vi "init_panel.vi"(6 "Run":refnum<vi>, 7 "Succesfull Run":refnum<vi>, 8 "Parameters Tree":refnum<vi>, 9 "Plot Tree":refnum<vi>, 10 "Spec File Loaded?":refnum<vi>, 11 "Vali File Loaded?":refnum<vi>) -> ()   [LabVIEW 2019]
uses:
  Biogas_LabView_Wrapper/lib/libBioGasLabViewWrapper.so
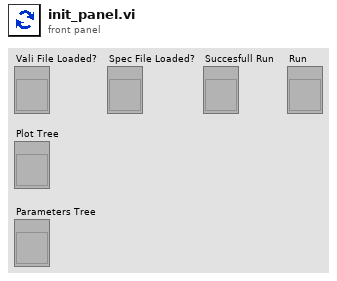
[diagram p1: front panel]
types:
  T1 = enum8{"Enabled", "Disabled", "Disabled and Grayed Out"}
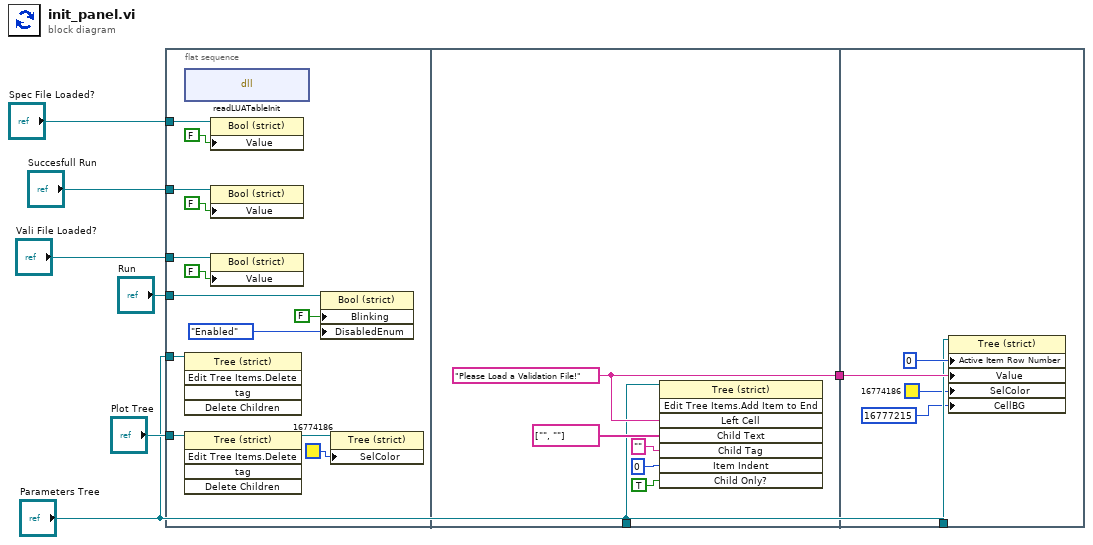
[diagram p0: block diagram]
diagram:
  n1 = flat-sequence {
    tunnel: "Vali File Loaded?" -> [w19]
    tunnel: "Plot Tree" -> [w18]
    tunnel: "Parameters Tree" -> [w17]
    tunnel: "Spec File Loaded?" -> [w16]
    tunnel: "Succesfull Run" -> [w14]
    tunnel: "Run" -> [w12]
    tunnel: [w23] -> w7
    tunnel: "Parameters Tree" -> [w21]
    tunnel: w7 -> [w30]
    tunnel: "Parameters Tree" -> [w29]
    frame #0 {
      n2 = dll-call lib="home/paul/Schreibtisch/Biogas_LabView_Wrapper/lib/libBioGasLabViewWrapper.so" fn="readLUATableInit"() -> ()  [unwired: 4 in, 2 out]
      n3 = invoke on="Invoke Node" class="Tree (strict)" method="Edit Tree Items.Delete"(reference=w17) -> ()  [unwired: 4 in, 5 out]
      n4 = invoke on="Invoke Node" class="Tree (strict)" method="Edit Tree Items.Delete"(reference=w18) -> (reference out=w9:refnum<vi>)  [unwired: 4 in, 4 out]
      n5 = property class="Bool (strict)"(reference=w16, "Value"=FALSE) -> ()  [unwired: 1 in, 2 out]
      n6 = property class="Bool (strict)"(reference=w14, "Value"=FALSE) -> ()  [unwired: 1 in, 2 out]
      n7 = property class="Bool (strict)"(reference=w19, "Value"=FALSE ("Vali File Loaded")) -> ()  [unwired: 1 in, 2 out]
      n8 = property class="Bool (strict)"(reference=w12, "Blinking"=FALSE, "DisabledEnum"=T1."Enabled" ("Disabled")) -> ()  [unwired: 1 in, 2 out]
      n9 = property class="Tree (strict)"(reference=w9, "SelColor"=u32 16774186) -> ()  [unwired: 1 in, 2 out]
    }
    frame #1 {
      w23 = "Please Load a Validation File!" ("Parent Tag")
      n10 = invoke on="Invoke Node" class="Tree (strict)" method="Edit Tree Items.Add Item to End"(reference=w21, "Left Cell"=w23, "Child Text"=string[] ["", ""], "Child Tag"="", "Item Indent"=0 ("New Item Indentation"), "Child Only?"=TRUE) -> ()  [unwired: 2 in, 8 out]
    }
    frame #2 {
      n11 = property on="Property Node" class="Tree (strict)"(reference=w29, "Active Item Row Number"=0 ("Active Item:Row Number"), "Value"=w30, "SelColor"=u32 16774186, "CellBG"=u32 16777215 ("Active Cell:Background Color")) -> ()  [unwired: 1 in, 2 out]
    }
  }
